vi "配置文件路径.vi"(8 "error in (no error)":errorcluster caption="错误输入（无错误）", 11 "Cleaningcycle 输入":refnum<class "Cleaning cycle.lvclass">) -> (0 "error out":errorcluster caption="错误输出", 3 "Cleaningcycle 输出":refnum<class "Cleaning cycle.lvclass">)   [LabVIEW 2022 SP3, in "Cleaning cycle.lvclass"]
uses:
  Cleaning cycle.lvclass
  Cleaning cycle.lvclass/Cleaning cycle.ctl
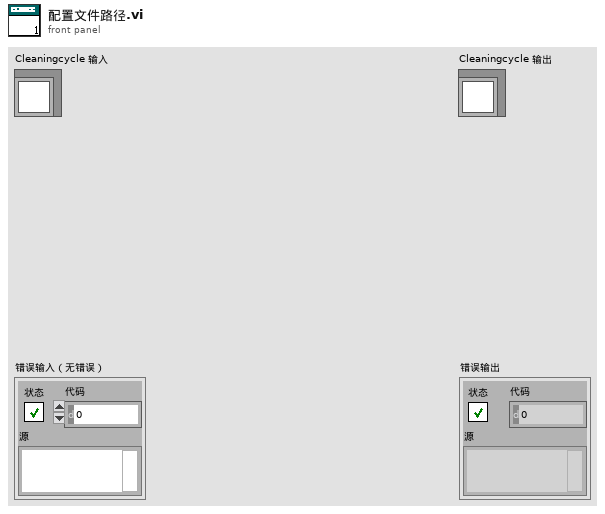
[diagram p1: front panel]
types:
  T1 = typedef "Cleaning cycle.lvclass/State Data.ctl" = cluster{"配置文件路径":path, "简易流程路径":path, "参数列表":cluster{"String":string, "Value":u16}[], "简易流程列表":cluster{"String":string, "Value":u16}[], "配置信息":T2, "命令":cluster{"触发":bool, "周期项":T4}[]}
  T2 = typedef "Cleaning cycle.lvclass/配置信息.ctl" = cluster{"任务列表":T3}
  T3 = typedef "Cleaning cycle.lvclass/任务.ctl" = cluster{"启用":bool, "项":string[][]}
  T4 = typedef "Cleaning cycle.lvclass/周期项.ctl" = cluster{"时":i32, "分":i32, "频次":string, "id":i32, "参数":string, "simpleflowid":i32, "简易流程名称":string}
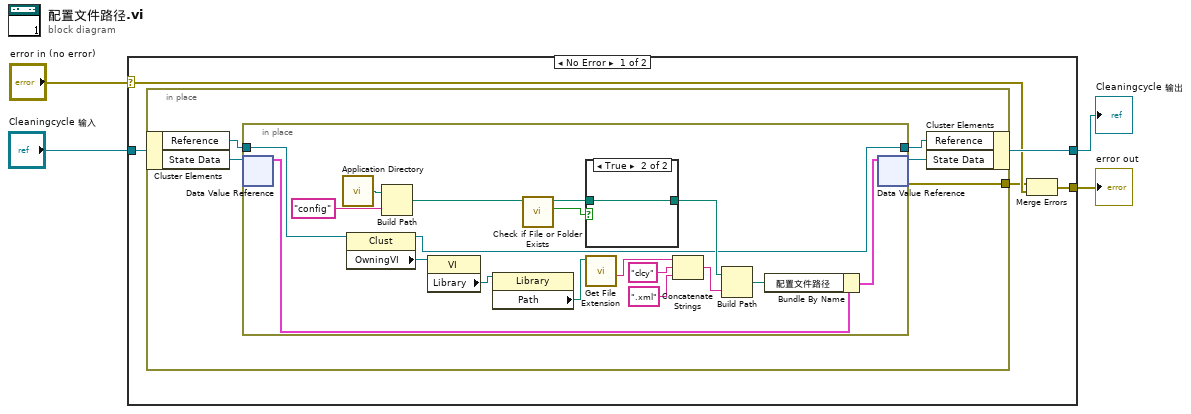
[diagram p0: block diagram]
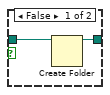
[diagram p2: hidden frame]
diagram:
  n1 = case shown="No Error" "error in (no error)" {
    selector: "error in (no error)" -> [w7 w37]
    tunnel: [w5 w37] -> w3
    tunnel: [w8 w36] -> w1
    tunnel: "Cleaningcycle 输入" -> [w9 w36]
    frame No Error {
      n2 = in-place {
        in-place-border: [w10] -> w6
        n3 = in-place-cluster #1(w9) -> ("Reference"=w14:refnum<vi>, "State Data"=w12:refnum<data-value>)
        n4 = in-place {
          in-place-border: w14 -> [w21]
          in-place-border: [w20] -> w13
          n5 = in-place-dvr #2(w12) -> (w19:T1)  [unwired: 1 out]
          n6 = call <vilib>:"Application Directory.vi"() -> ("Application Directory"=w29:path)
          n7 = property class="Clust"(reference=w21) -> (reference out=w20:refnum<vi>, "OwningVI"=w31:refnum<vi>)  [unwired: 1 in, 1 out]
          n8 = Build Path(base path=w29, name or relative path="config" ("名称或相对路径")) -> (appended path=w27:path)
          n9 = property class="VI"(reference=w31) -> ("Library"=w32:refnum<vi>)  [unwired: 1 in, 2 out]
          n10 = property class="Library"(reference=w32) -> ("Path"=w30:path)  [unwired: 1 in, 2 out]
          n11 = call <vilib>:"Check if File or Folder Exists.vi"("path"=w27) -> ("file or folder exists?"=w24:bool, "dup path"=w23:path)  [unwired: 8 in, 1 out]
          n12 = case shown="True" w24 {
            tunnel: w23 -> [w34 w35]
            tunnel: [w33 w35] -> w22
            frame False {
              n13 = Create Folder(path (use dialog)=w34) -> (created path=w33:path)  [unwired: 2 in, 2 out]
            }
            frame True {
            }
          }
          n14 = call <vilib>:"Get File Extension.vi"("file"=w30) -> ("filename without extension"=w16:string)  [unwired: 6 in, 4 out]
          n15 = Concatenate Strings(w16, "clcy" ("字符串"), ".xml" ("字符串")) -> (w25:string)
          n16 = Build Path(base path=w22, name or relative path=w25) -> (appended path=w17:path)
          n17 = Bundle By Name(cluster=w19, "配置文件路径"=w17) -> (w18:T1)
          n18 = in-place-dvr #2(w18) -> (w11:refnum<data-value>, w10:errorcluster)
        }
        n19 = in-place-cluster #1("Reference"=w13, "State Data"=w11) -> (w8:refnum<class "Cleaning cycle.lvclass">)
      }
      n20 = Merge Errors(w6, w7) -> (w5:errorcluster)
    }
    frame Error {
    }
  }
  "error out" <- w3
  "Cleaningcycle 输出" <- w1
